vi "niRFUtil CONV Complex WDT to Complex Waveform.vi"(7 "Complex WDT":T1) -> (8 "Complex Waveform":T2 {"y" format="%.2f"; "dx" format="%^.2e"; "x0" format="%^.2e"})   [LabVIEW 2015, in "niRFUtil.lvlib"]
uses:
  niRFUtil.lvlib
  Includes/niRFUtil INC Complex Waveform.ctl
  Includes/niRFUtil INC Complex Array.ctl
  Includes/niRFUtil INC Complex WDT.ctl
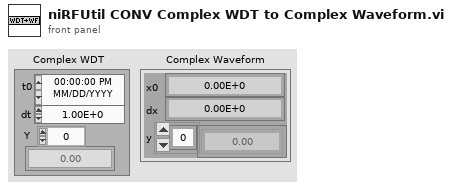
[diagram p1: front panel]
types:
  T1 = typedef "niRFUtil.lvlib/niRFUtil INC Complex WDT.ctl" = waveform(csg)
  T2 = typedef "niRFUtil.lvlib/niRFUtil INC Complex Waveform.ctl" = cluster{"x0":dbl, "dx":dbl, "y":T3}
  T3 = typedef "niRFUtil.lvlib/niRFUtil INC Complex Array.ctl" = csg[]
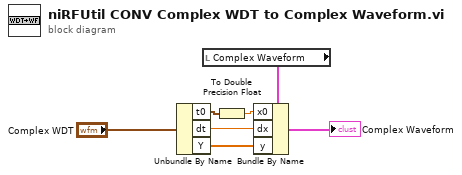
[diagram p0: block diagram]
diagram:
  n1 = Unbundle By Name("Complex WDT") -> ("t0"=w4:timestamp, "dt"=w6:dbl, "Y"=w5:csg[])
  n2 = local read "Complex Waveform"() -> (w1:T2)
  n3 = To Double Precision Float(number=w4) -> (double precision float=w3:dbl)
  n4 = Bundle By Name(cluster=w1, "x0"=w3, "dx"=w6, "y"=w5) -> (→"Complex Waveform":T2)
